vi "Write Timestamp.vi"(7 "field name":string="timeStamp", 8 "error in":errorcluster, 9 "user tag":i32, 10 "timestamp":timestamp, 11 "Value in":refnum<class "Value.lvclass">) -> (0 "error out":errorcluster, 3 "Value out":refnum<class "Value.lvclass">)   [LabVIEW 2020, in "Value.lvlib" / "Value.lvclass"]
uses:
  Value.lvclass
  Value.lvclass/Value.ctl
  Value.lvlib
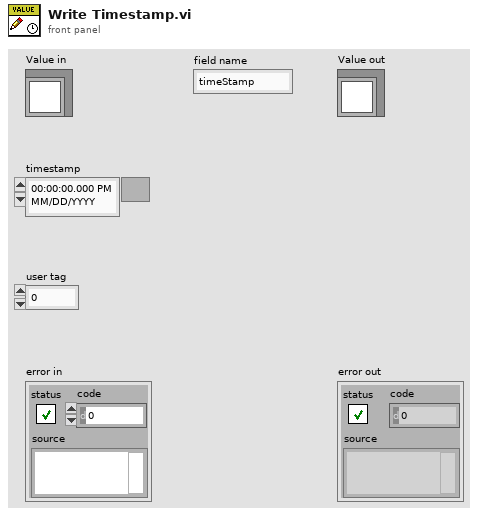
[diagram p1: front panel]
types:
  T1 = typedef "Value.lvlib/Timestamp.ctl" = cluster{"Seconds Past Epoch":i64, "Nanoseconds":i32, "User Tag":i32}
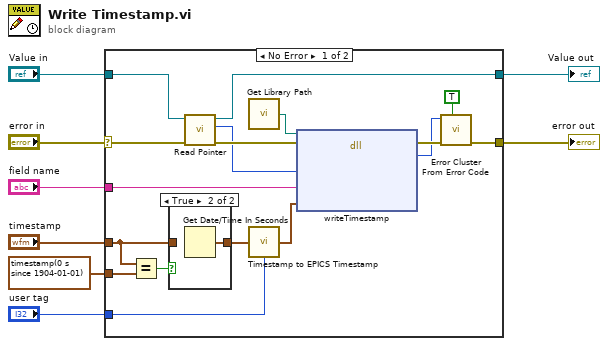
[diagram p0: block diagram]
diagram:
  n1 = case shown="No Error" "error in" {
    selector: "error in" -> [w20 w29]
    tunnel: [w21 w29] -> w8
    tunnel: "Value in" -> [w18 w28]
    tunnel: [w16 w28] -> w5
    tunnel: "field name" -> [w15 _]
    tunnel: "timestamp" -> [w12 _]
    tunnel: "user tag" -> [w10 _]
    tunnel: timestamp(0 s since 1904-01-01) ("timestamp 2") -> [w14 _]
    frame No Error {
      n2 = Equal?(x=w12, y=w14) -> (x = y?=w13:bool)
      n3 = case shown="True" w13 {
        tunnel: [w26 w27] -> w11
        tunnel: w12 -> [w26 _]
        frame False {
        }
        frame True {
          n4 = Get Date/Time In Seconds() -> (seconds since 1Jan1904=w27:timestamp)
        }
      }
      n5 = call-dynamic "Read Pointer.vi"("error in (no error)"=w20, "Value in"=w18) -> ("error out"=w19:errorcluster, "pointer"=w17:i64, "Value out"=w16:refnum<class "Value.lvclass">)  [unwired: 7 in]
      n6 = call "Get Library Path.vi"() -> ("Path"=w25:path)  [unwired: 1 in]
      n7 = call "Timestamp to EPICS Timestamp.vi"("timestamp"=w11, "user tag"=w10) -> ("epics timestamp"=w9:T1)
      n8 = dll-call lib="?" fn="writeTimestamp"(path in=w25, error in=w19, "value"=w17, "field_name"=w15, "timestamp"=w9) -> (error out=w23:errorcluster, "err_code"=w22:i32)  [unwired: 4 in, 1 out]
      n9 = call <vilib>:"Error Cluster From Error Code.vi"("show call chain? (False)"=TRUE, "error in (no error)"=w23, "error code (0)"=w22) -> ("error out"=w21:errorcluster)  [unwired: 6 in]
    }
    frame Error {
    }
  }
  "error out" <- w8
  "Value out" <- w5
